vi "FTW-Package-Request-WriteResponse.vi"(8 "error in":errorcluster, 9 "Response Body":string, 11 "FTW Incoming Request":refnum<class "FTW-Package-IncomingRequest.lvclass">) -> (0 "error out":errorcluster, 3 "FTW Incoming Request out":refnum<class "FTW-Package-IncomingRequest.lvclass">)   [LabVIEW 2013, in "FTW-Package-IncomingRequest.lvclass"]
uses:
  FTW-Package-IncomingRequest.lvclass
  FTW-Package-IncomingRequest.lvclass/FTW-Package-IncomingRequest.ctl
panel:
  # "Inputs"
  # "Outputs"
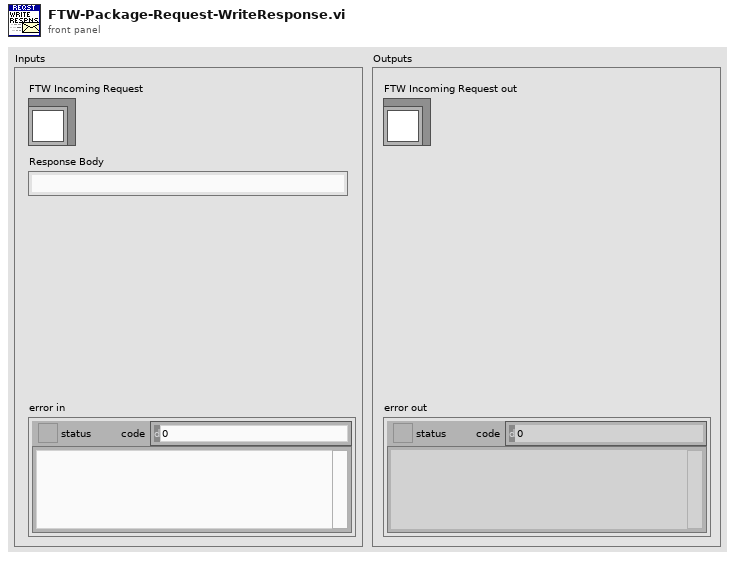
[diagram p1: front panel]
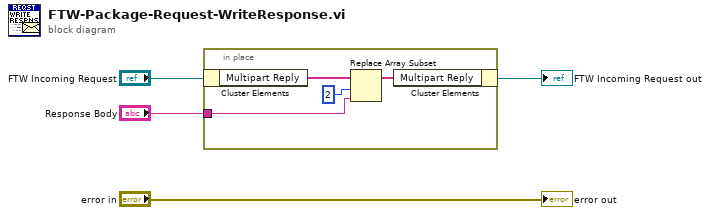
[diagram p0: block diagram]
diagram:
  n1 = in-place {
    in-place-border: "Response Body" -> [w5]
    n2 = in-place-cluster #1("FTW Incoming Request") -> ("Multipart Reply"=w8:string[])
    n3 = Replace Array Subset(array=w8, new element=w5, index=2) -> (w7:string[])
    n4 = in-place-cluster #1("Multipart Reply"=w7) -> (→"FTW Incoming Request out":refnum<class "FTW-Package-IncomingRequest.lvclass">)
  }
  "error out" <- "error in"
